vi "Keithley 2450 Read Single.vi"() -> ()   [LabVIEW 2020]
doc: "This example shows how to configure a measurement and take a reading."
uses:
  <instrlib>/Keithley 2450/Keithley 2450.lvlib
panel:
  in  "Output Level (0)":dbl
  in  "Compliance Level (0.1)":dbl=0.1
  in  "error in (no error)":errorcluster
  in  "Source Mode  (0: Voltage)":u16(ring) items=["Voltage", "Current"]
  out "Resistance (ohm)":dbl
  out "Current (A)":dbl
  out "Voltage (V)":dbl
  in  "VISA resource name":refnum<visa-resource-name>
  # "(c) 2006 National Instruments.  ALL RIGHTS RESERVED."
  # "(c) 2021 National Instruments.  ALL RIGHTS RESERVED."
  # "Source Settings"
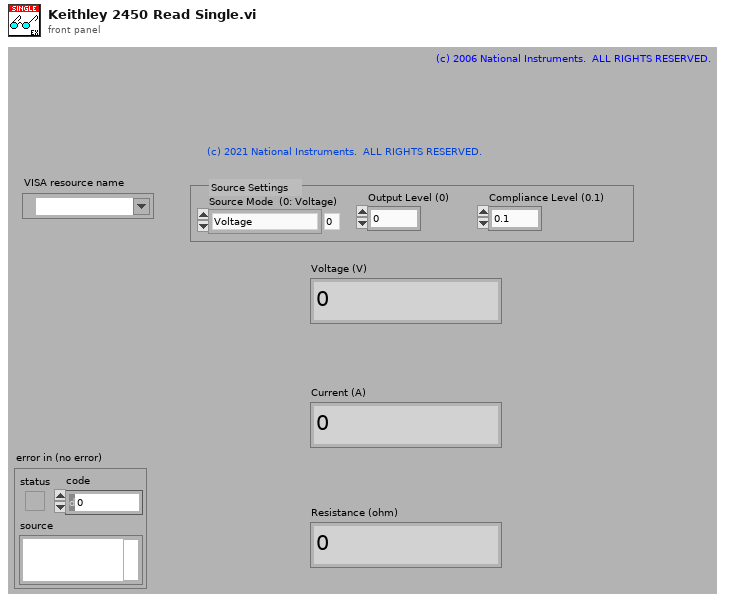
[diagram p1: front panel]
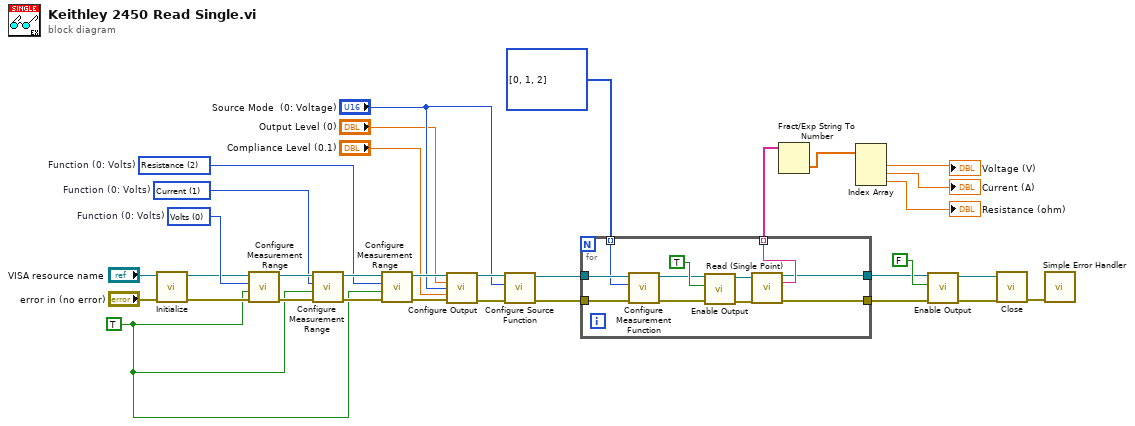
[diagram p0: block diagram]
diagram:
  w3 = TRUE ("Enable Output (T: Enable)")
  w9 = u16[] [0, 1, 2] items=["Volts", "Current", "Auto Resistance"]
  w25 = u16 2 items=["Volts", "Current", "Resistance"]  # Function (0: Volts)
  w26 = u16 1 items=["Volts", "Current", "Resistance"]  # Function (0: Volts)
  w27 = u16 0 items=["Volts", "Current", "Resistance"]  # Function (0: Volts)
  n1 = call <instrlib>:"Initialize.vi"("error in (no error)"="error in (no error)", "VISA resource name"="VISA resource name") -> ("error out"=w20:errorcluster, "VISA resource name out"=w21:refnum<visa-resource-name>)  [unwired: 8 in]
  n2 = call <instrlib>:"Configure Measurement Range.vi"("error in (no error)"=w20, "Enable Auto Range (T:Enable)"=w3, "Function (0: Volts)"=w27, "VISA resource name"=w21) -> ("error out"=w30:errorcluster, "VISA resource name out"=w31:refnum<visa-resource-name>)  [unwired: 6 in]
  n3 = call <instrlib>:"Configure Measurement Range.vi"("error in (no error)"=w30, "Enable Auto Range (T:Enable)"=w3, "Function (0: Volts)"=w26, "VISA resource name"=w31) -> ("error out"=w29:errorcluster, "VISA resource name out"=w28:refnum<visa-resource-name>)  [unwired: 6 in]
  n4 = call <instrlib>:"Configure Measurement Range.vi"("error in (no error)"=w29, "Enable Auto Range (T:Enable)"=w3, "Function (0: Volts)"=w25, "VISA resource name"=w28) -> ("error out"=w23:errorcluster, "VISA resource name out"=w22:refnum<visa-resource-name>)  [unwired: 6 in]
  n5 = call <instrlib>:"Configure Output.vi"("VISA resource name"=w22, "Source Level (0)"="Output Level (0)", "Source Mode  (0: Voltage)"="Source Mode  (0: Voltage)", "Source Limit Level (0.1)"="Compliance Level (0.1)", "error in (no error)"=w23) -> ("VISA resource name out"=w8:refnum<visa-resource-name>, "error out"=w7:errorcluster)  [unwired: 9 in]
  n6 = call <instrlib>:"Configure Source Function.vi"("error in (no error)"=w7, "Function (0: Volts)"="Source Mode  (0: Voltage)", "VISA resource name"=w8) -> ("error out"=w6:errorcluster, "VISA resource name out"=w5:refnum<visa-resource-name>)  [unwired: 7 in]
  n7 = for {
    tunnel: w5 -> [w44]
    tunnel: w6 -> [w43]
    tunnel: [w42] -> w14 mode=indexing
    tunnel: [w41] -> w16
    tunnel: [w40] -> w15
    tunnel: w9 -> [w39] mode=indexing
    n8 = call <instrlib>:"Configure Measurement Function.vi"("error in (no error)"=w43, "Function (0: Volts)"=w39, "VISA resource name"=w44) -> ("error out"=w36:errorcluster, "VISA resource name out"=w37:refnum<visa-resource-name>)  [unwired: 7 in]
    n9 = call <instrlib>:"Enable Output.vi"("error in (no error)"=w36, "Enable Output (T: Enable)"=TRUE, "VISA resource name"=w37) -> ("error out"=w35:errorcluster, "VISA resource name out"=w34:refnum<visa-resource-name>)  [unwired: 7 in]
    n10 = call <instrlib>:"Read (Single Point).vi"("VISA resource name"=w34, "error in (no error)"=w35) -> ("VISA resource name out"=w41:refnum<visa-resource-name>, "Data out"=w42:string, "error out"=w40:errorcluster)  [unwired: 11 in]
  }
  n11 = Fract/Exp String To Number(string=w14) -> (number=w13:dbl[])  [unwired: 3 in, 1 out]
  n12 = Index Array(array=w13) -> (element #1=→"Voltage (V)":dbl, element #2=→"Current (A)":dbl, element #3=→"Resistance (ohm)":dbl)  [unwired: 3 in]
  n13 = call <instrlib>:"Enable Output.vi"("error in (no error)"=w15, "Enable Output (T: Enable)"=FALSE, "VISA resource name"=w16) -> ("error out"=w17:errorcluster, "VISA resource name out"=w18:refnum<visa-resource-name>)  [unwired: 7 in]
  n14 = call <instrlib>:"Close.vi"("error in (no error)"=w17, "VISA resource name"=w18) -> ("error out"=w33:errorcluster)  [unwired: 9 in]
  n15 = call <vilib>:"Simple Error Handler.vi"("error in (no error)"=w33) -> ()  [unwired: 4 in, 5 out]
